vi "ReactorSIM.vi"() -> ()   [LabVIEW 2018]
uses:
  <vilib>/Simulation/Scripting/Companion Diagram/SimConfigNode/SimParams.ctl
  <vilib>/Simulation/Scripting/Companion Diagram/SimConfigNode/_simSolvers.ctl
  <vilib>/Simulation/Implementation/Shared/SIMSCR Execution Mode.ctl
  <vilib>/Simulation/Param Hierarchy/Typedefs/SIMPH Param Control Actions.ctl
  <vilib>/Simulation/Implementation/Shared/SIM limit type.ctl
  <vilib>/Simulation/Scripting/Editor Utilities/SIM subVI tag data.ctl
  <vilib>/Simulation/Scripting/Editor Utilities/SIM subVI execution type.ctl
  <vilib>/Simulation/Implementation/Shared/NILVSim_ParamChanged.vi
  <vilib>/Simulation/Implementation/Shared/NILVSIM_BeginStep.vi
  <vilib>/Simulation/Utility/Implementation/SIM Halt.vi
  <vilib>/Simulation/Utility/Implementation/SIM Time.vi
  <vilib>/Simulation/ContinuousLinear/Implementation/NILVSim Integrator new.llb/SIM Integrator distributor (scalar).vi
  <vilib>/Simulation/SignalDisplay/Implementation/NILVSim Time Waveform.llb/SIM Time Waveform (scalar).vi
  <vilib>/Simulation/Implementation/Shared/SIM Fire Discrete SubVI.vi
  <vilib>/Simulation/ContinuousLinear/Implementation/NILVSim Integrator new.llb/SIM Integrator collector (scalar).vi
  <vilib>/Simulation/Implementation/Shared/NILVSim_Manager.vi
  <vilib>/Utility/error.llb/Clear Errors.vi
  <vilib>/Simulation/Implementation/Shared/NILVSim_FinalizeModel.vi
  <vilib>/Simulation/Implementation/Shared/SIM Fire Discrete SubVI (Core).vi
  <vilib>/Simulation/Implementation/Shared/SIM Unbundle Sim Info.vi
  <vilib>/Simulation/Implementation/Shared/NILVSim_Initialize.vi
  <vilib>/imath/engines/lvmath2/RunTimeEngine/Managers/WorkSpace/UID Generator.vi
  <vilib>/imath/engines/lvmath2/RunTimeEngine/RunTimeType/NIMS_RunTimeType_From StrictType (excl LVString).vi
  <instcachedir>/0/NIMS_RunTimeType_From StrictType (excl LVString)_E7E34A65C99947108168652BAD14964D.lvgen/NIMS_RunTimeType_From StrictType (excl LVString)_E7E34A65C99947108168652BAD14964D_000.vi
  <vilib>/imath/engines/lvmath2/RunTimeEngine/LocalVariableDefStatement/MC_LocalVariableDefStatement_Display.vi
  <vilib>/imath/engines/lvmath2/RunTimeEngine/Managers/SymbolTable/Clear UID.vi
  <vilib>/imath/engines/lvmath2/RunTimeEngine/NodeEndStatement/NIMS_NodeEndStatement_Output.vi
  <instcachedir>/0/NIMS_NodeEndStatement_Output_53EC0D466D134D7ABD903AC30B43404B.lvgen/NIMS_NodeEndStatement_Output_53EC0D466D134D7ABD903AC30B43404B_001.vi
  <vilib>/imath/engines/lvmath2/RunTimeEngine/ErrorHandling/NIMS_Finalize Error.vi
  <instcachedir>/0/NIMS_NodeEndStatement_Output_53EC0D466D134D7ABD903AC30B43404B.lvgen/NIMS_NodeEndStatement_Output_53EC0D466D134D7ABD903AC30B43404B_009.vi
  <vilib>/Simulation/Utility/Implementation/NILVSim Get Time and IsAcceptedStep.vi
  <instcachedir>/0/NIMS_NodeEndStatement_Output_53EC0D466D134D7ABD903AC30B43404B.lvgen/NIMS_NodeEndStatement_Output_53EC0D466D134D7ABD903AC30B43404B_010.vi
  Sig-Override.vi
  <vilib>/Simulation/Implementation/Shared/SIMSH Read Queue.vi
  <vilib>/Simulation/Implementation/Shared/NILVSim_GetModelError.vi
  <vilib>/Simulation/Implementation/Shared/SIM Bundle Sim Info.vi
  <vilib>/Simulation/Scripting/Companion Diagram/SimConfigNode/SimDog.xnode
  <vilib>/Simulation/Implementation/XNodeFramework/SimXNode/SimX.xnode
  <vilib>/Simulation/ContinuousLinear/Implementation/NILVSim Integrator new.llb/SIM Integrator (scalar).vi
  <vilib>/imath/engines/lvmath2/RunTimeEngine/Managers/SymbolTable/NIMS_WorkSpace.lvlib
  <vilib>/Simulation/Implementation/Shared/NI_SIM_Implementation.lvlib
panel:
  out "Cooling Water Temperature":waveform(dbl)(graph)
  out "Reactor Temperature":waveform(dbl)(graph)
  out "Reactor Concentration":waveform(dbl)(graph)
  out "Reactor Level":waveform(dbl)(graph)
  in  "BPCS-SIM-RX-ARRAY":dbl[](array[numeric])=[50.0, 50.0, 50.0]
  out "appended array":dbl[](array[numeric])
  in  "SIM Parameters":T1={"Step Size (s)"=0.01, "Final Time (s)"=700.0, "ODE Solver"=enum."Runge-Kutta 4"}
  in  "Valve CV":cluster{"Cv":dbl, "Cv0":dbl, "CvJ":dbl}={"Cv"=4.0, "Cv0"=4.0, "CvJ"=12.336}
  in  "Reactor Disturbances":cluster{"T0":dbl, "CA0":dbl, "TJ0":dbl}={"T0"=323.0, "CA0"=2.0, "TJ0"=300.0}
  in  "Reactor Parameters":T2={"E_R"=8330.1, "A"=1.3, "Lam"=130000000.0, "Alpha"=10000000000.0, "rho"=1000000.0, "rhoj"=1000000.0, "Cp"=1.0, "CJ"=1.0, "U_AH"=1678000.0, "VJ"=10.0} {"U_AH" format="%#_6e"; "rhoj" format="%#_6e"; "rho" format="%#_6e"; "Alpha" format="%#_6e"; "Lam" format="%#_6e"}
  in  "Halt?":bool
  out "simulation time":dbl=5.2700000000000005
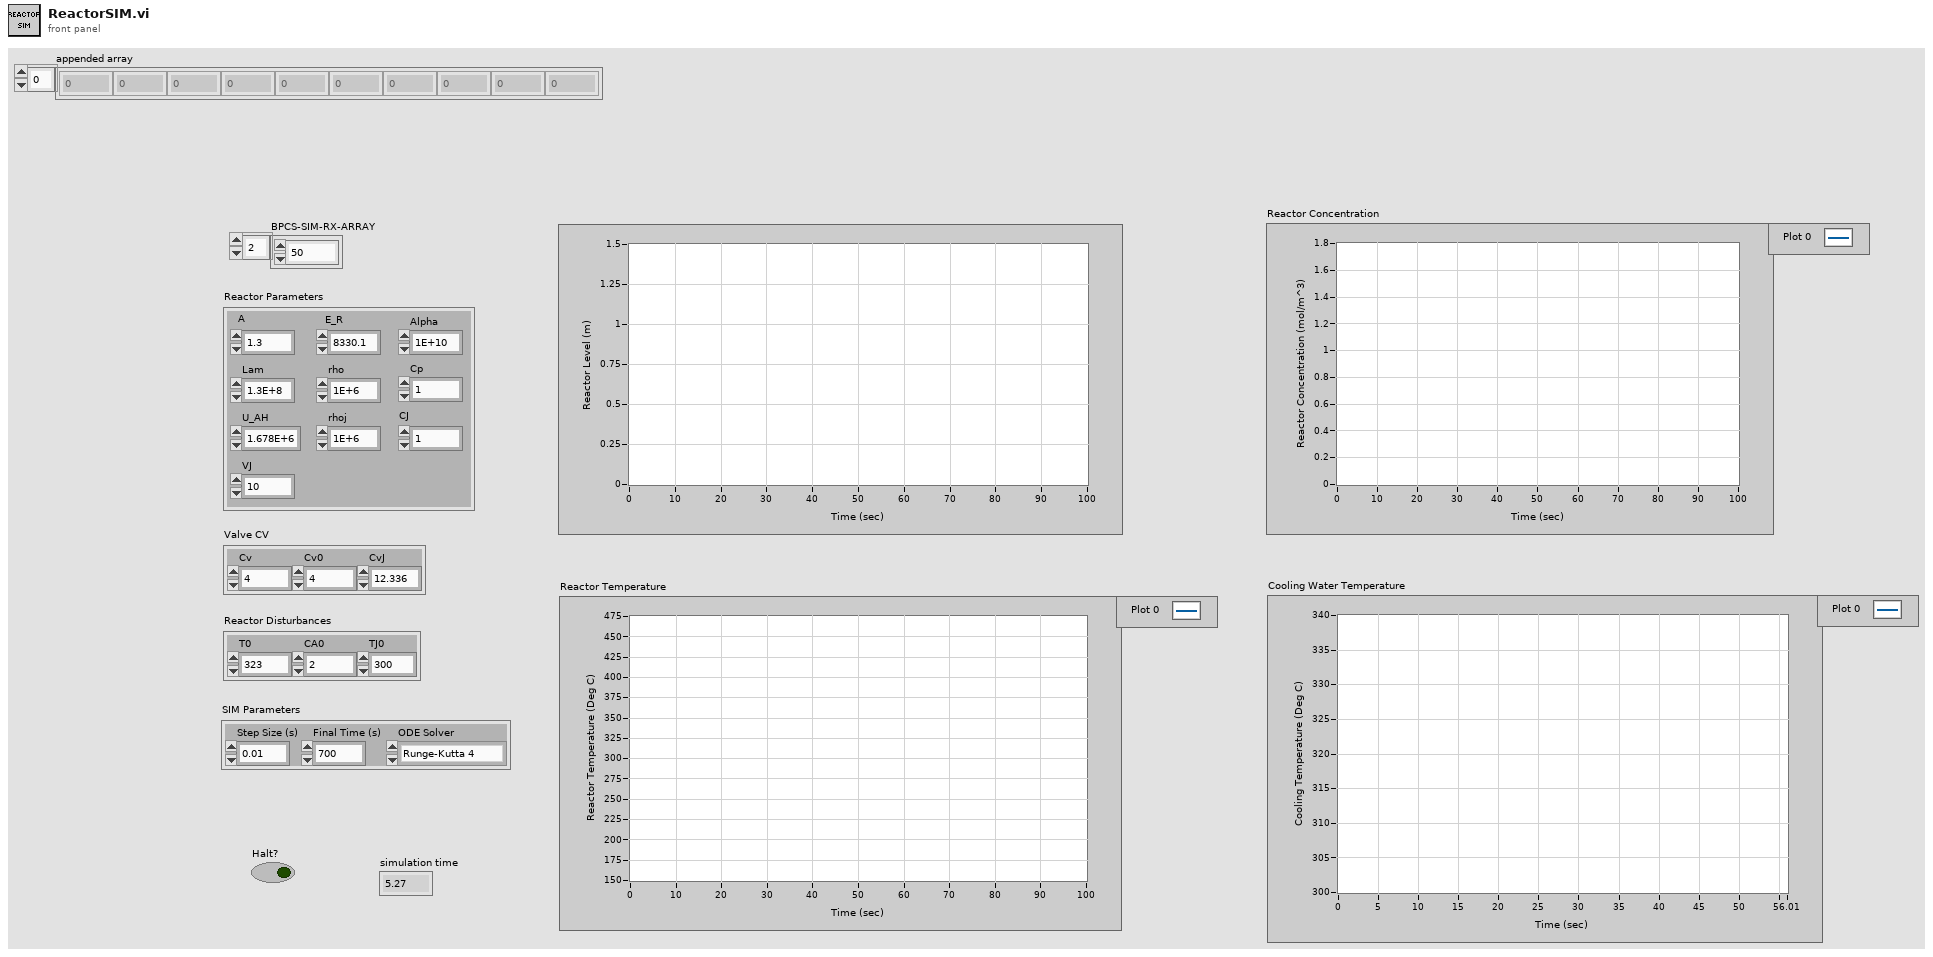
[diagram p1: front panel]
types:
  T1 = cluster{"Step Size (s)":dbl, "Final Time (s)":dbl, "ODE Solver":enum16{"Runge-Kutta 1 (Euler)", "Runge-Kutta 2", "Runge-Kutta 3", "Runge-Kutta 4", "Runge-Kutta 23 (variable)", "Runge-Kutta 45 (variable)", "BDF (variable)", "Adams-Moulton (variable)", "Rosenbrock (variable)", "Discrete States Only", "SDIRK 4 (variable)", "Radau 5 (variable)", "Radau 9 (variable)", "Radau 13 (variable)", "Radau [Variable Order] (variable)", "Gear's Method (variable)"}}
  T2 = cluster{"E_R":dbl, "A":dbl, "Lam":dbl, "Alpha":dbl, "rho":dbl, "rhoj":dbl, "Cp":dbl, "CJ":dbl, "U_AH":dbl, "VJ":dbl}
  T3 = enum16{"Runge-Kutta 1 (Euler)", "Runge-Kutta 2", "Runge-Kutta 3", "Runge-Kutta 4", "Runge-Kutta 23 (variable)", "Runge-Kutta 45 (variable)", "BDF (variable)", "Adams-Moulton (variable)", "Rosenbrock (variable)", "Discrete States Only", "SDIRK 4 (variable)", "Radau 5 (variable)", "Radau 9 (variable)", "Radau 13 (variable)", "Radau [Variable Order] (variable)", "Gear's Method (variable)"}
  T4 = typedef "imagedata.ctl" = cluster{"image type":i32, "image depth":i32, "image":u8[], "mask":u8[], "colors":u32[], "Rectangle":cluster{"left":i16, "top":i16, "right":i16, "bottom":i16}}
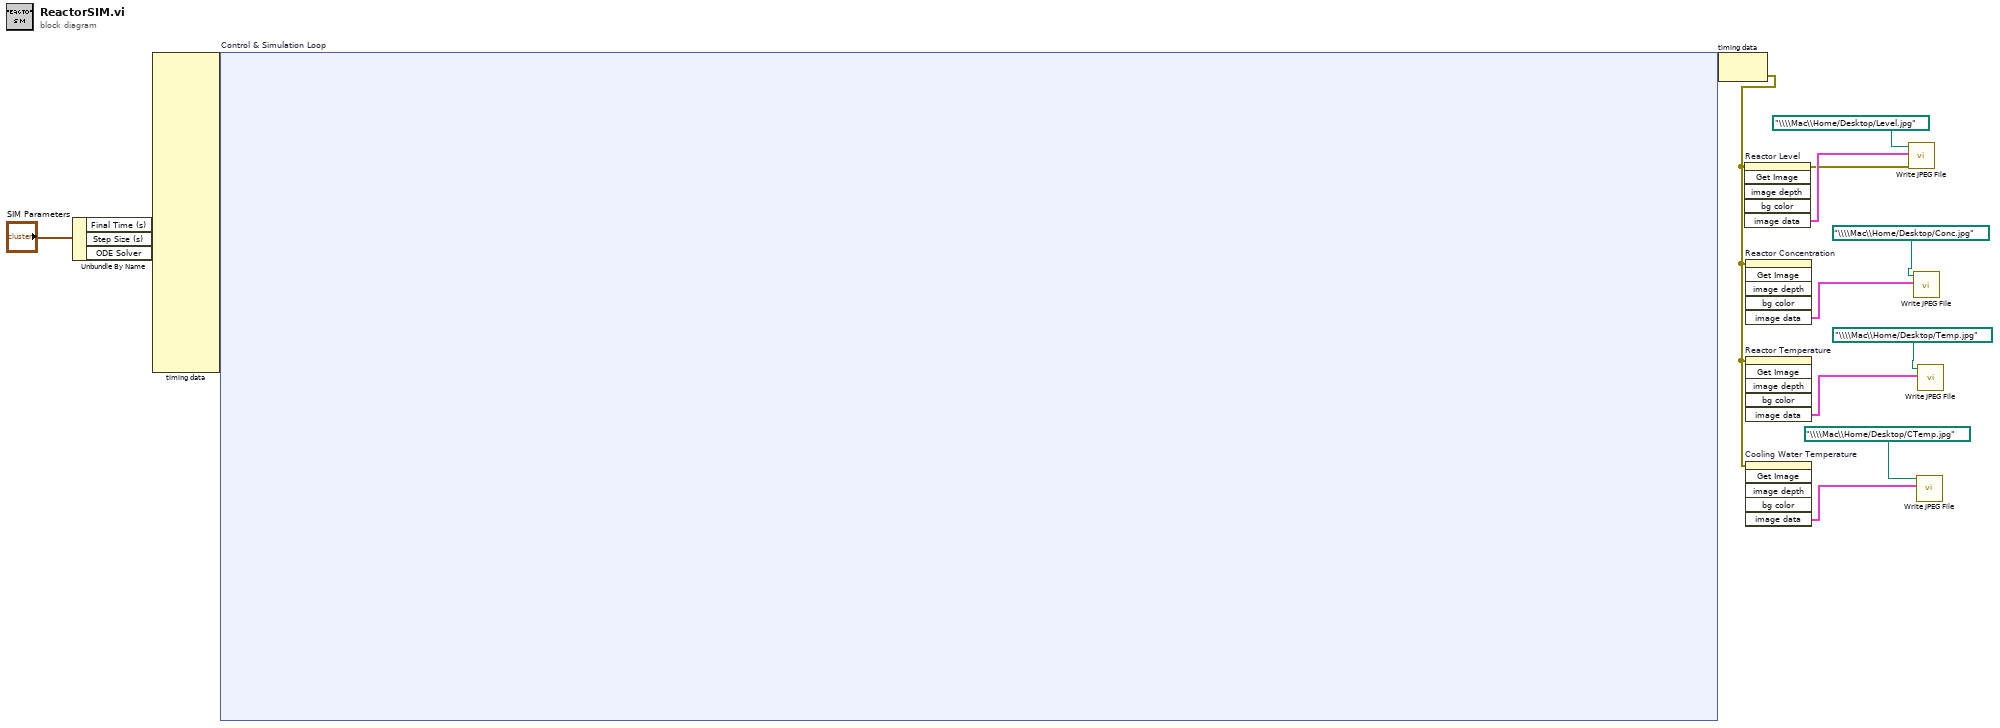
[diagram p0: block diagram]
diagram:
  n1 = Unbundle By Name ("Unbundle By Name 3")("SIM Parameters") -> ("Final Time (s)"=w12:dbl, "Step Size (s)"=w13:dbl, "ODE Solver"=w14:T3)
  n2 = node-c288(w12, w13, w14) -> (w16:variant)  [unwired: 21 in]
  n3 = node-c254 "Control & Simulation Loop"(w16) -> (w15:variant)
  n4 = node-c288(w15) -> (w1:errorcluster)
  n5 = invoke on="Reactor Level" class="WFChart (strict)" method="Get Image"(error in=w1) -> (error out=w8:errorcluster, "image data"=w9:T4)  [unwired: 5 in, 4 out]
  n6 = invoke on="Reactor Concentration" class="WFChart (strict)" method="Get Image"(error in=w1) -> ("image data"=w7:T4)  [unwired: 5 in, 5 out]
  n7 = invoke on="Reactor Temperature" class="WFChart (strict)" method="Get Image"(error in=w1) -> ("image data"=w4:T4)  [unwired: 5 in, 5 out]
  n8 = invoke on="Cooling Water Temperature" class="WFChart (strict)" method="Get Image"(error in=w1) -> ("image data"=w3:T4)  [unwired: 5 in, 5 out]
  n9 = call <vilib>:"Write JPEG File.vi"("error in (no error)"=w8, "image data"=w9, "path to JPEG file"=path "\\\\Mac\\Home/Desktop/Level.jpg") -> ()  [unwired: 7 in, 2 out]
  n10 = call <vilib>:"Write JPEG File.vi"("image data"=w7, "path to JPEG file"=path "\\\\Mac\\Home/Desktop/Conc.jpg") -> ()  [unwired: 8 in, 2 out]
  n11 = call <vilib>:"Write JPEG File.vi"("image data"=w3, "path to JPEG file"=path "\\\\Mac\\Home/Desktop/CTemp.jpg") -> ()  [unwired: 8 in, 2 out]
  n12 = call <vilib>:"Write JPEG File.vi"("image data"=w4, "path to JPEG file"=path "\\\\Mac\\Home/Desktop/Temp.jpg") -> ()  [unwired: 8 in, 2 out]
